vi "AOD controller Sarah.vi"() -> ()   [LabVIEW 2010]
uses:
  <vilib>/DAQmx/write.llb/DAQmx Write (Analog DBL 1Chan 1Samp).vi
  <vilib>/DAQmx/create/channels.llb/DAQmx Create Channel (AO-Voltage-Basic).vi
  <vilib>/daqmx/miscellaneous.llb/DAQmx Fill In Error Info.vi
  <vilib>/Utility/inputDevices.llb/keyboardAcquire.vi
panel:
  in  "Laser Power":dbl format="%0.2f"
  in  "Laser":bool
  in  "stop":bool
  in  "frequency":i32=20
  in  "Speed XY":dbl=1.0 min=0.0 max=20.0
  in  "Speed Z":dbl=1.0 min=0.0 max=20.0
  out "Y (-1000-1000)":dbl=-6372.0
  out "X  (-600-7000) 8":dbl=7095.0
  out "Z  (7 in - 9 out)":dbl=-378.0
  in  "Reset":bool
  in  "switch":bool
  in  "Motors":bool=TRUE
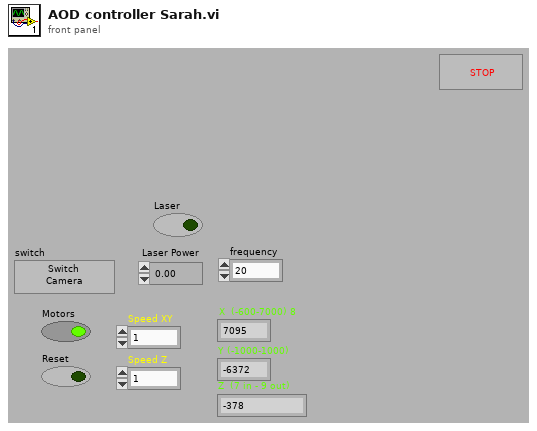
[diagram p1: front panel]
types:
  T1 = enum16{"0", "1", "2", "3", "4", "5", "6", "7", "8", "9", "A", "B", "C", "D", "E", "F", "G", "H", "I", "J", "K", "L", "M", "N", "O", "P", "Q", "R", "S", "T", "U", "V", "W", "X", "Y", "Z", "F1", "F2", "F3", "F4", "F5", "F6", "F7", "F8", "F9", "F10", "F11", "F12", "F13", "F14", "F15", "ADD", "BACK", "BACKSLASH", "CAPITAL", "COMMA", "DECIMAL", "DELETE", "DIVIDE", "DOWN", "END", "EQUALS", "ESCAPE", "GRAVE (`)", "HOME", "INSERT", "LBRACKET", "LCONTROL", "LEFT", "L ALT", "LSHIFT", "LWIN", "MINUS", "MULTIPLY", "NEXT", "NUMLOCK", "NUMPAD_0", "NUMPAD_1", "NUMPAD_2", "NUMPAD_3", "NUMPAD_4", "NUMPAD_5", "NUMPAD_6", "NUMPAD_7", "NUMPAD_8", "NUMPAD_9", "PAUSE", "PERIOD", "PRIOR (PG UP)", "RBRACKET", "RCONTROL", "RETURN", "RIGHT", "R ALT", "RSHIFT", "RWIN", "SCROLL", "SEMICOLON", "SLASH", "SPACE", "SUBTRACT", "TAB", "UP", "ENTER (num pad)", "' (quote)"}[]
  T2 = enum16{"0", "1", "2", "3", "4", "5", "6", "7", "8", "9", "A", "B", "C", "D", "E", "F", "G", "H", "I", "J", "K", "L", "M", "N", "O", "P", "Q", "R", "S", "T", "U", "V", "W", "X", "Y", "Z", "F1", "F2", "F3", "F4", "F5", "F6", "F7", "F8", "F9", "F10", "F11", "F12", "F13", "F14", "F15", "ADD", "BACK", "BACKSLASH", "CAPITAL", "COMMA", "DECIMAL", "DELETE", "DIVIDE", "DOWN", "END", "EQUALS", "ESCAPE", "GRAVE (`)", "HOME", "INSERT", "LBRACKET", "LCONTROL", "LEFT", "L ALT", "LSHIFT", "LWIN", "MINUS", "MULTIPLY", "NEXT", "NUMLOCK", "NUMPAD_0", "NUMPAD_1", "NUMPAD_2", "NUMPAD_3", "NUMPAD_4", "NUMPAD_5", "NUMPAD_6", "NUMPAD_7", "NUMPAD_8", "NUMPAD_9", "PAUSE", "PERIOD", "PRIOR (PG UP)", "RBRACKET", "RCONTROL", "RETURN", "RIGHT", "R ALT", "RSHIFT", "RWIN", "SCROLL", "SEMICOLON", "SLASH", "SPACE", "SUBTRACT", "TAB", "UP", "ENTER (num pad)", "' (quote)"}
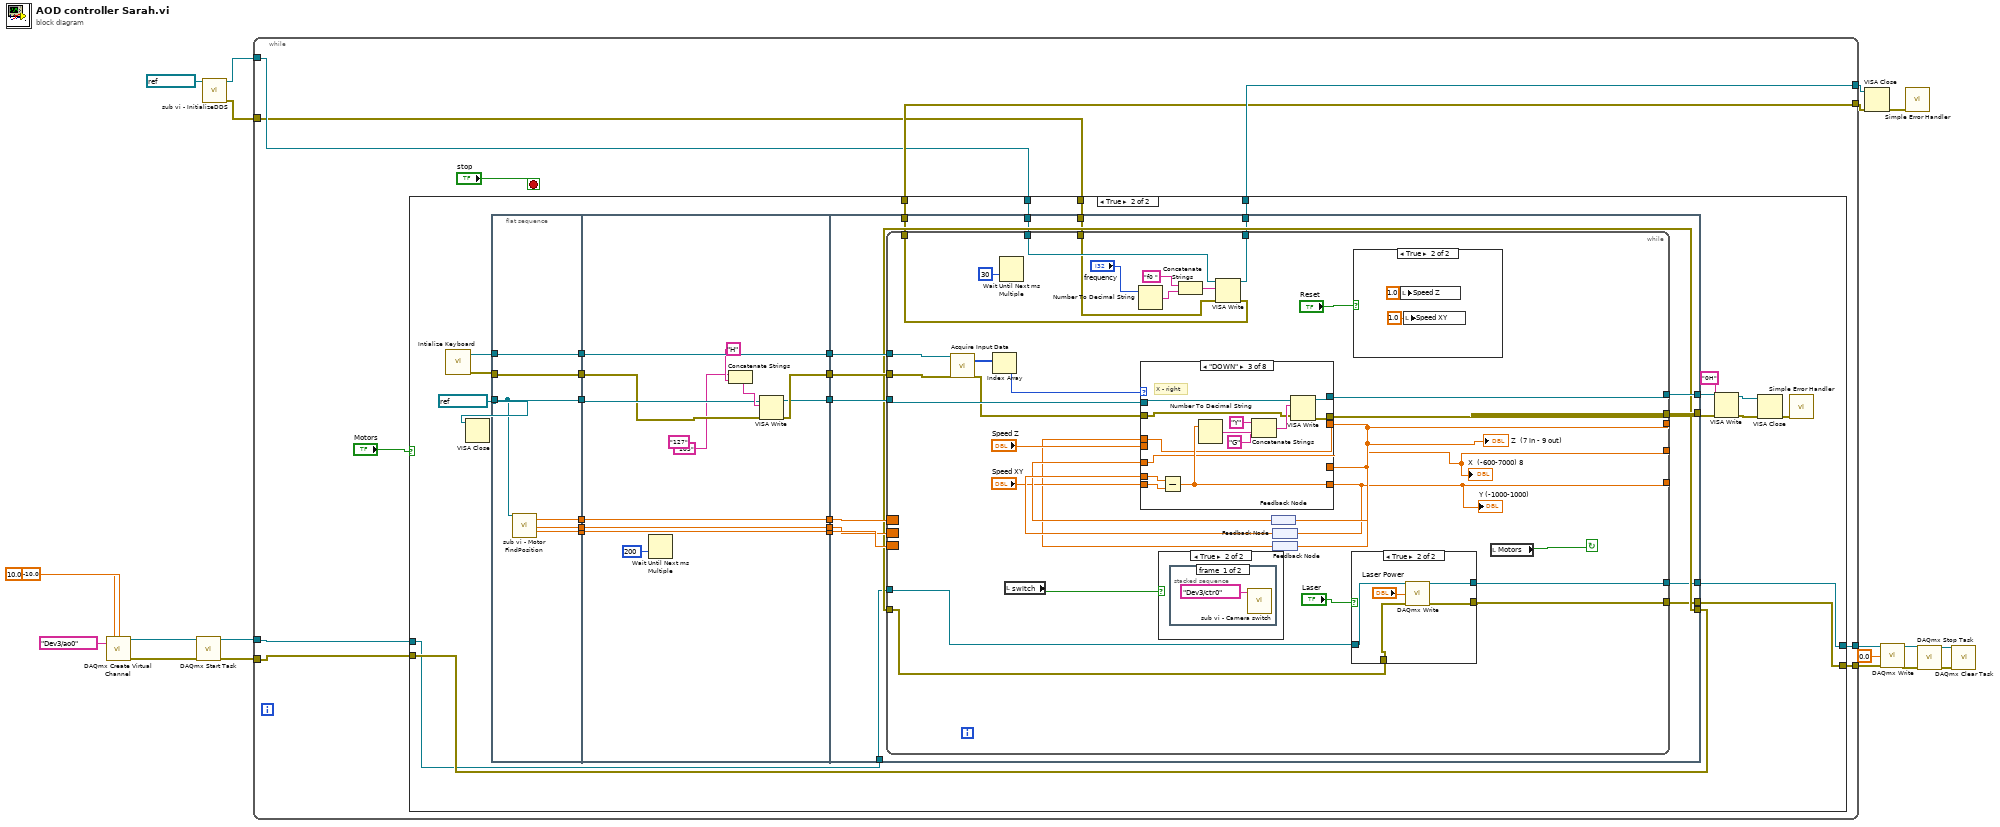
[diagram p0: block diagram]
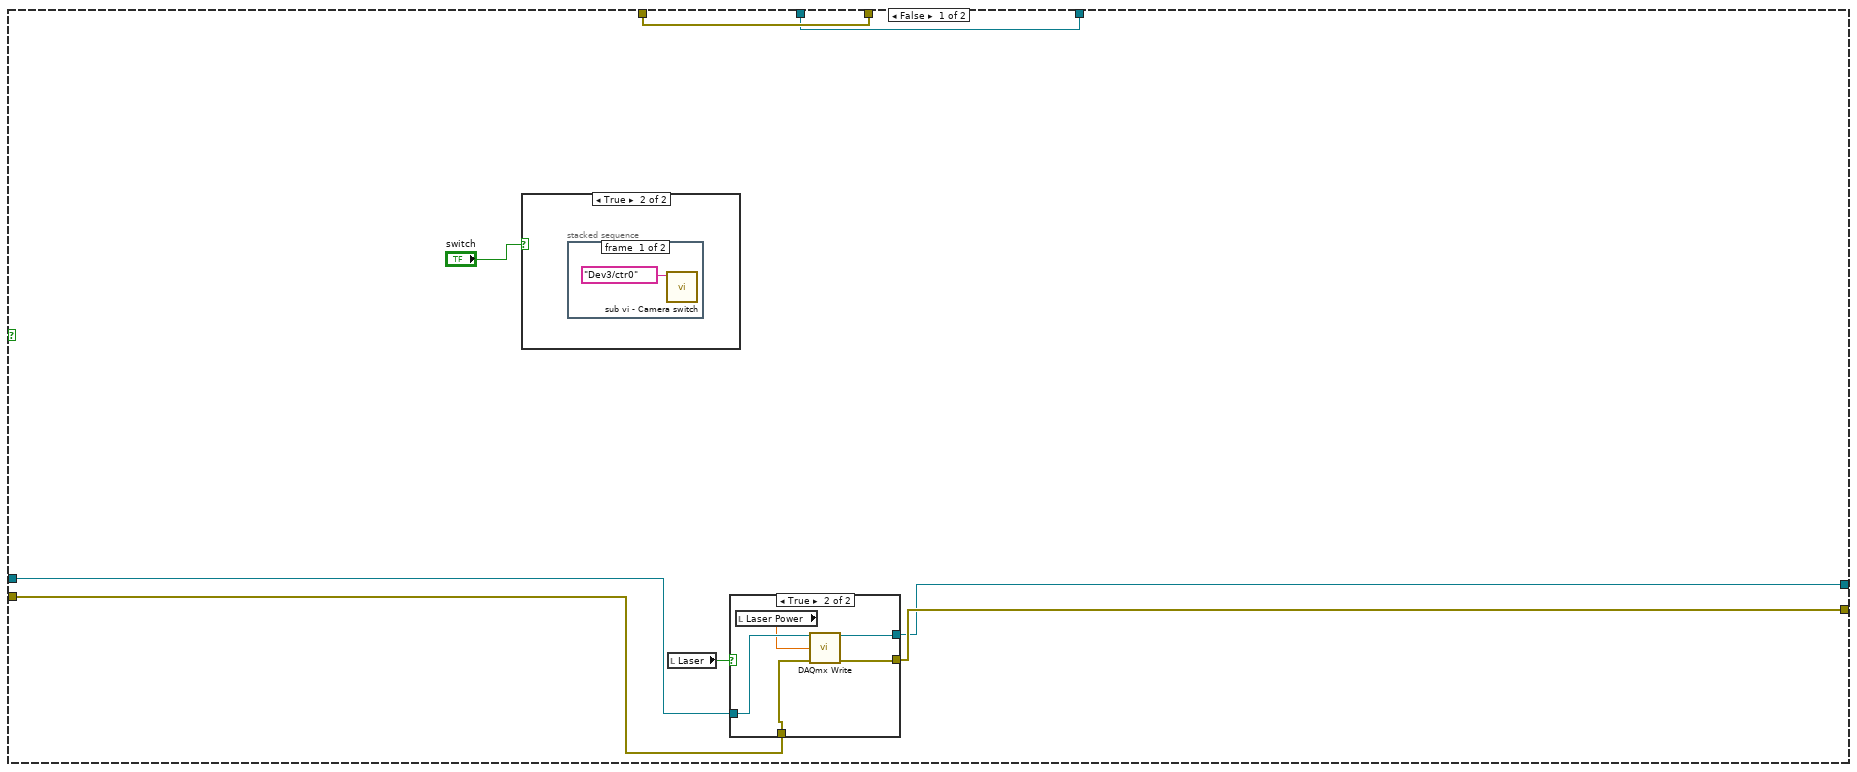
[diagram p2: hidden frame]
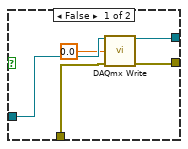
[diagram p3: hidden frame]
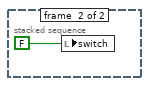
[diagram p5: hidden frame]
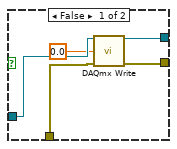
[diagram p6: hidden frame]
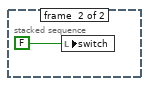
[diagram p9: hidden frame]
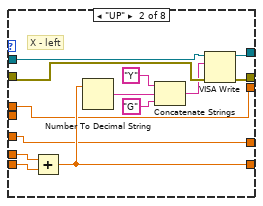
[diagram p11: hidden frame]
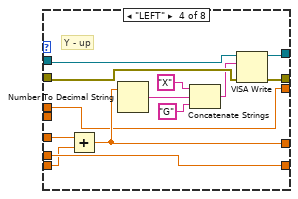
[diagram p12: hidden frame]
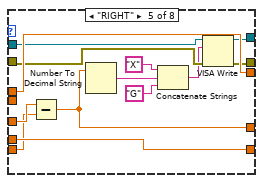
[diagram p13: hidden frame]
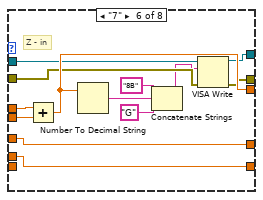
[diagram p14: hidden frame]
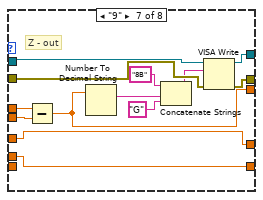
[diagram p15: hidden frame]
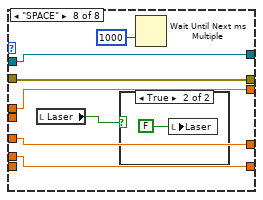
[diagram p16: hidden frame]
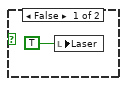
[diagram p17: hidden frame]
diagram:
  n1 = call-poly <vilib>:"DAQmx Create Virtual Channel.vi"("maximum value"=10.0, "minimum value"=-10.0, "physical channels"=tag "Dev3/ao0") -> ("task out"=w18:refnum<k21>, "error out"=w17:errorcluster)  [unwired: 6 in, 5 out]
  n2 = call <vilib>:"DAQmx Start Task.vi"("task/channels in"=w18, "error in"=w17) -> ("task out"=w15:refnum<k21>, "error out"=w16:errorcluster)  [unwired: 12 out]
  n3 = call "sub vi - InitializeDDS.vi"("VISA resource name"=refnum<visa-resource-name> "COM19") -> ("error out"=w6:errorcluster, "reference out"=w7:refnum<visa-resource-name>)  [unwired: 8 in, 1 out]
  n4 = while {
    tunnel: w15 -> [w28]
    tunnel: w16 -> [w27]
    tunnel: w7 -> [w22]
    tunnel: w6 -> [w21]
    tunnel: [w23] -> w5
    tunnel: [w24] -> w4
    tunnel: [w26] -> w3
    tunnel: [w25] -> w2
    stop <- "stop" stop-if-true
    n5 = case shown="True" "Motors" {
      tunnel: w28 -> [w37 w57]
      tunnel: w27 -> [w36 w58]
      tunnel: [w34 w56] -> w26
      tunnel: [w35 w55] -> w25
      tunnel: [w31 w54] -> w24
      tunnel: [w32 w53] -> w23
      tunnel: w22 -> [w31 w52]
      tunnel: w21 -> [w32 w51]
      frame False {
        n6 = case shown="True" "switch" {
          frame False {
          }
          frame True {
            n7 = stacked-sequence {
              frame #0 {
                n8 = call "sub vi - Camera switch.vi"("Counter"=tag "Dev3/ctr0") -> ()  [unwired: 11 out]
              }
              frame #1 {
                n9 = local write "switch"(FALSE ("Switch Camera")) -> ()
              }
            }
          }
        }
        n10 = local read "Laser"() -> (w33:bool)
        n11 = case shown="True" w33 {
          tunnel: w37 -> [w40 w48]
          tunnel: w36 -> [w41 w47]
          tunnel: [w43 w46] -> w34
          tunnel: [w42 w45] -> w35
          frame False {
            n12 = call-poly <vilib>:"DAQmx Write.vi"("task/channels in"=w40, "data"=0.0, "error in"=w41) -> ("task out"=w43:refnum<k21>, "error out"=w42:errorcluster)  [unwired: 1 in, 10 out]
          }
          frame True {
            n13 = local read "Laser Power"() -> (w44:dbl)
            n14 = call-poly <vilib>:"DAQmx Write.vi"("task/channels in"=w48, "data"=w44, "error in"=w47) -> ("task out"=w46:refnum<k21>, "error out"=w45:errorcluster)  [unwired: 1 in, 10 out]
          }
        }
      }
      frame True {
        w59 = refnum<visa-resource-name> "COM30" ("bottom (large beads)")
        n15 = call <vilib>:"Intialize Keyboard.vi"() -> ("error out"=w67:errorcluster, "device ID"=w66:refnum<k1>)  [unwired: 1 in, 9 out]
        n16 = VISA Close(VISA resource name=w59) -> ()  [unwired: 1 in, 1 out]
        n17 = flat-sequence {
          tunnel: w59 -> [w80]
          tunnel: w66 -> [w84]
          tunnel: w67 -> [w85]
          tunnel: [w85] -> w79
          tunnel: [w84] -> w78
          tunnel: [w80] -> w77
          tunnel: [w81] -> w76
          tunnel: [w83] -> w75
          tunnel: [w82] -> w74
          tunnel: [w97] -> w73
          tunnel: [w96] -> w72
          tunnel: [w95] -> w71
          tunnel: [w94] -> w70
          tunnel: [w90] -> w69
          tunnel: [w89] -> w68
          tunnel: w79 -> [w87]
          tunnel: w78 -> [w97]
          tunnel: w77 -> [w88]
          tunnel: w76 -> [w96]
          tunnel: w75 -> [w95]
          tunnel: w74 -> [w94]
          tunnel: [w108] -> w63
          tunnel: w73 -> [w113]
          tunnel: w72 -> [w111]
          tunnel: w71 -> [w110]
          tunnel: w70 -> [w109]
          tunnel: w69 -> [w107]
          tunnel: [w106] -> w64
          tunnel: w68 -> [w112]
          tunnel: w58 -> [w105]
          tunnel: w57 -> [w104]
          tunnel: [w103] -> w56
          tunnel: [w102] -> w55
          tunnel: [w101] -> w54
          tunnel: [w100] -> w53
          tunnel: w52 -> [w99]
          tunnel: w51 -> [w98]
          frame #0 {
            n18 = call "sub vi - Motor FindPosition.vi"("VISA resource name"=w80) -> ("X"=w83:dbl, "Y"=w82:dbl, "Z"=w81:dbl)  [unwired: 6 in, 10 out]
          }
          frame #1 {
            (unwired) "127" ("string")
            n19 = Wait Until Next ms Multiple(millisecond multiple=u32 200) -> ()  [unwired: 1 out]
            n20 = Concatenate Strings("105" ("string"), "H" ("string")) -> (w91:string)
            n21 = VISA Write(VISA resource name=w88, write buffer=w91, error in (no error)=w87) -> (VISA resource name out=w89:refnum<visa-resource-name>, error out=w90:errorcluster)  [unwired: 1 out]
          }
          frame #2 {
            n22 = while {
              tunnel: w107 -> [w146]
              tunnel: w113 -> [w145]
              tunnel: [w128] -> _
              tunnel: [w129] -> _
              border: w109 -> [_]
              border: w110 -> [_]
              border: w111 -> [_]
              tunnel: w112 -> [w138]
              tunnel: [w132] -> _
              tunnel: [w135] -> w108
              tunnel: [w134] -> w106
              tunnel: w105 -> [w125]
              tunnel: w104 -> [w126]
              tunnel: [w124] -> w103
              tunnel: [w123] -> w102
              tunnel: [w117] -> w101
              tunnel: [w116] -> w100
              tunnel: w99 -> [w115]
              tunnel: w98 -> [w114]
              stop <- w127 continue-if-true
              n23 = call-poly <vilib>:"Acquire Input Data.vi"("device ID"=w145, "error in (no error)"=w146) -> ("keys pressed"=w143:T1, "error out"=w133:errorcluster)  [unwired: 16 out]
              n24 = Index Array(array=w143) -> (element=w139:T2)  [unwired: 1 in]
              n25 = Wait Until Next ms Multiple(millisecond multiple=u32 30) -> ()  [unwired: 1 out]
              n26 = local read "switch"() -> (w131:bool)
              n27 = Number To Decimal String(number="frequency") -> (decimal integer string=w119:string)  [unwired: 1 out]
              n28 = case shown="True" w131 {
                frame False {
                }
                frame True {
                  n29 = stacked-sequence {
                    frame #0 {
                      n30 = call "sub vi - Camera switch.vi"("Counter"=tag "Dev3/ctr0") -> ()  [unwired: 11 out]
                    }
                    frame #1 {
                      n31 = local write "switch"(FALSE ("Switch Camera")) -> ()
                    }
                  }
                }
              }
              n32 = Concatenate Strings("f0 " ("string"), w119) -> (w120:string)
              n33 = VISA Write(VISA resource name=w115, write buffer=w120, error in (no error)=w114) -> (VISA resource name out=w117:refnum<visa-resource-name>, error out=w116:errorcluster)  [unwired: 1 out]
              n34 = feedback #1() -> (w141:dbl)
              n35 = feedback #2() -> (w142:dbl)
              n36 = feedback #3() -> (w136:dbl)
              n37 = case shown="\"DOWN\"" w139 {
                tunnel: w142 -> [w165 w175 w191 w199 w212 w223 w236 w246]
                tunnel: [w165 w173 w190 w199 w212 w223 w236 w246] -> w128
                tunnel: w141 -> [w164 w172 w186 w201 w214 w224 w237 w247]
                tunnel: [w164 w172 w186 w200 w213 w224 w237 w247] -> w129
                tunnel: "Speed XY" -> [_ w174 w185 w197 w210 _ _ _]
                tunnel: w138 -> [w162 w167 w183 w196 w209 w222 w235 w250]
                tunnel: "Speed Z" -> [_ _ _ _ _ w226 w239 _]
                tunnel: w136 -> [w163 w171 w184 w198 w211 w225 w240 w248]
                tunnel: [w163 w171 w184 w198 w211 w227 w238 w248] -> w132
                tunnel: [w161 w169 w179 w194 w207 w220 w233 w249] -> w135
                tunnel: [w162 w170 w182 w195 w208 w219 w234 w250] -> w134
                tunnel: w133 -> [w161 w168 w180 w193 w206 w221 w232 w249]
                frame "0", Default {
                }
                frame "UP" {
                  # "X - left"
                  n38 = Add(x=w175, y=w174) -> (x+y=w173:dbl)
                  n39 = Number To Decimal String(number=w173) -> (decimal integer string=w178:string)  [unwired: 1 out]
                  n40 = Concatenate Strings("Y", w178, "G") -> (w166:string)
                  n41 = VISA Write(VISA resource name=w167, write buffer=w166, error in (no error)=w168) -> (VISA resource name out=w170:refnum<visa-resource-name>, error out=w169:errorcluster)  [unwired: 1 out]
                }
                frame "DOWN" {
                  # "X - right"
                  n42 = Subtract(x=w191, y=w185) -> (x-y=w190:dbl)
                  n43 = Number To Decimal String(number=w190) -> (decimal integer string=w189:string)  [unwired: 1 out]
                  n44 = Concatenate Strings("Y", w189, "G") -> (w181:string)
                  n45 = VISA Write(VISA resource name=w183, write buffer=w181, error in (no error)=w180) -> (VISA resource name out=w182:refnum<visa-resource-name>, error out=w179:errorcluster)  [unwired: 1 out]
                }
                frame "LEFT" {
                  # "Y - up"
                  n46 = Add(x=w201, y=w197) -> (x+y=w200:dbl)
                  n47 = Number To Decimal String(number=w200) -> (decimal integer string=w202:string)  [unwired: 1 out]
                  n48 = Concatenate Strings("X", w202, "G") -> (w192:string)
                  n49 = VISA Write(VISA resource name=w196, write buffer=w192, error in (no error)=w193) -> (VISA resource name out=w195:refnum<visa-resource-name>, error out=w194:errorcluster)  [unwired: 1 out]
                }
                frame "RIGHT" {
                  n50 = Subtract(x=w214, y=w210) -> (x-y=w213:dbl)
                  n51 = Number To Decimal String(number=w213) -> (decimal integer string=w217:string)  [unwired: 1 out]
                  n52 = Concatenate Strings("X", w217, "G") -> (w205:string)
                  n53 = VISA Write(VISA resource name=w209, write buffer=w205, error in (no error)=w206) -> (VISA resource name out=w208:refnum<visa-resource-name>, error out=w207:errorcluster)  [unwired: 1 out]
                }
                frame "7" {
                  # "Z - in"
                  n54 = Add(x=w225, y=w226) -> (x+y=w227:dbl)
                  n55 = Number To Decimal String(number=w227) -> (decimal integer string=w230:string)  [unwired: 1 out]
                  n56 = Concatenate Strings("8B", w230, "G") -> (w218:string)
                  n57 = VISA Write(VISA resource name=w222, write buffer=w218, error in (no error)=w221) -> (VISA resource name out=w219:refnum<visa-resource-name>, error out=w220:errorcluster)  [unwired: 1 out]
                }
                frame "9" {
                  # "Z - out"
                  n58 = Subtract(x=w240, y=w239) -> (x-y=w238:dbl)
                  n59 = Number To Decimal String(number=w238) -> (decimal integer string=w243:string)  [unwired: 1 out]
                  n60 = Concatenate Strings("8B", w243, "G") -> (w231:string)
                  n61 = VISA Write(VISA resource name=w235, write buffer=w231, error in (no error)=w232) -> (VISA resource name out=w234:refnum<visa-resource-name>, error out=w233:errorcluster)  [unwired: 1 out]
                }
                frame "SPACE" {
                  n62 = local read "Laser"() -> (w245:bool)
                  n63 = case shown="True" w245 {
                    frame False {
                      n64 = local write "Laser"(TRUE ("Boolean")) -> ()
                    }
                    frame True {
                      n65 = local write "Laser"(FALSE ("Boolean")) -> ()
                    }
                  }
                  n66 = Wait Until Next ms Multiple(millisecond multiple=u32 1000) -> ()  [unwired: 1 out]
                }
              }
              "Y (-1000-1000)" <- w128
              "X  (-600-7000) 8" <- w129
              "Z  (7 in - 9 out)" <- w132
              n67 = feedback-in #1(w129) -> ()
              n68 = feedback-in #2(w128) -> ()
              n69 = feedback-in #3(w132) -> ()
              n70 = case shown="True" "Laser" {
                tunnel: w126 -> [w148 w156]
                tunnel: w125 -> [w149 w155]
                tunnel: [w151 w154] -> w124
                tunnel: [w150 w153] -> w123
                frame False {
                  n71 = call-poly <vilib>:"DAQmx Write.vi"("task/channels in"=w148, "data"=0.0, "error in"=w149) -> ("task out"=w151:refnum<k21>, "error out"=w150:errorcluster)  [unwired: 1 in, 10 out]
                }
                frame True {
                  n72 = call-poly <vilib>:"DAQmx Write.vi"("task/channels in"=w156, "data"="Laser Power", "error in"=w155) -> ("task out"=w154:refnum<k21>, "error out"=w153:errorcluster)  [unwired: 1 in, 10 out]
                }
              }
              n73 = case shown="True" "Reset" {
                frame False {
                }
                frame True {
                  n74 = local write "Speed Z"(1.0 ("Speed Z")) -> ()
                  n75 = local write "Speed XY"(1.0 ("Speed XY")) -> ()
                }
              }
              n76 = local read "Motors"() -> (w127:bool)
            }
          }
        }
        n77 = VISA Write(VISA resource name=w64, write buffer="0H", error in (no error)=w63) -> (VISA resource name out=w61:refnum<visa-resource-name>, error out=w60:errorcluster)  [unwired: 1 out]
        n78 = VISA Close(VISA resource name=w61, error in (no error)=w60) -> (error out=w62:errorcluster)
        n79 = call <vilib>:"Simple Error Handler.vi"("error in (no error)"=w62) -> ()  [unwired: 1 in, 8 out]
      }
    }
  }
  n80 = VISA Close(VISA resource name=w4, error in (no error)=w5) -> (error out=w20:errorcluster)
  n81 = call-poly <vilib>:"DAQmx Write.vi"("task/channels in"=w3, "data"=0.0, "error in"=w2) -> ("task out"=w12:refnum<k21>, "error out"=w11:errorcluster)  [unwired: 1 in, 10 out]
  n82 = call <vilib>:"Simple Error Handler.vi"("error in (no error)"=w20) -> ()  [unwired: 1 in, 8 out]
  n83 = call <vilib>:"DAQmx Stop Task.vi"("task/channels in"=w12, "error in"=w11) -> ("task out"=w14:refnum<k21>, "error out"=w13:errorcluster)  [unwired: 12 out]
  n84 = call <vilib>:"DAQmx Clear Task.vi"("task in"=w14, "error in"=w13) -> ()  [unwired: 14 out]
